vi "Display Frame.vi"(8 "Error In":errorcluster, 10 "Frame":u32[][](array[colorbox]), 11 "Display In":refnum<class "Neopixel - RT.lvclass">) -> (0 "Error Out":errorcluster, 3 "Display Out":refnum<class "Neopixel - RT.lvclass">)   [LabVIEW 2021, in "Neopixel - RT.lvclass"]
uses:
  Neopixel - RT.lvclass
  Neopixel - RT.lvclass/Neopixel - RT.ctl
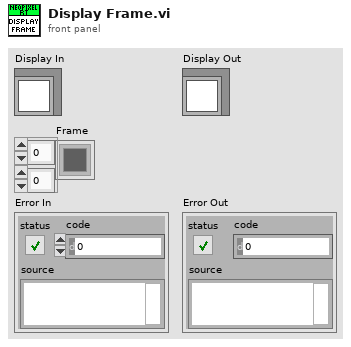
[diagram p1: front panel]
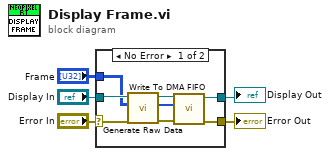
[diagram p0: block diagram]
diagram:
  n1 = case shown="No Error" "Error In" {
    selector: "Error In" -> [w10 w14]
    tunnel: "Display In" -> [w11 w15]
    tunnel: [w13 w14] -> w3
    tunnel: [w12 w15] -> w2
    tunnel: "Frame" -> [w9 _]
    frame No Error {
      n2 = call "Generate Raw Data.vi"("Error In"=w10, "Matrix"=w9, "Display In"=w11) -> ("Error Out"=w7:errorcluster, "Raw Data"=w6:u8[], "Display Out"=w8:refnum<class "Neopixel - RT.lvclass">)  [unwired: 6 in]
      n3 = call "Write To DMA FIFO.vi"("Error In"=w7, "Data"=w6, "Display In"=w8) -> ("Error Out"=w13:errorcluster, "Display Out"=w12:refnum<class "Neopixel - RT.lvclass">)  [unwired: 7 in]
    }
    frame Error {
    }
  }
  "Error Out" <- w3
  "Display Out" <- w2
